vi "take CRT data.vi"() -> ()   [LabVIEW 2016]
panel:
  out "File switch":bool
  out "Save CRT data":bool
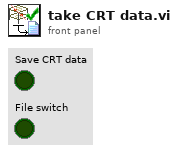
[diagram p1: front panel]
diagram:
